vi "dfd_CIC Decimation Simu.vi"(0 "signal in":i32[](array[numeric]), 1 "lag":i32, 2 "#stage":i32, 3 "init? (T)":bool, 5 "factor":i32, 7 "Acc width":i32[](array[numeric]), 9 "MSB pos":i16, 11 "FXPMRateSimState in":T1, 12 "Output wl":i16, 13 "q_mode":T3=enum."Truncation" caption="rounding mode", 14 "phase":i32) -> (4 "signal out":i32[](array[numeric]), 15 "FXPMRateSimState out":T1)   [LabVIEW 2017, in "NI_DigFilter_FXP.lvlib"]
uses:
  <vilib>/addons/Digital Filter Design/NI_DigFilter_FXP.lvlib
  <vilib>/addons/Digital Filter Design/_Objects.llb/DFD Round-off Mode.ctl
  <vilib>/addons/Digital Filter Design/_Objects.llb/dfd_FXP MRate Simu State.ctl
  <vilib>/addons/Digital Filter Design/_Objects.llb/dfd_Integer I160.ctl
  <vilib>/addons/Digital Filter Design/NI_DigFilterLicensed.lvlib
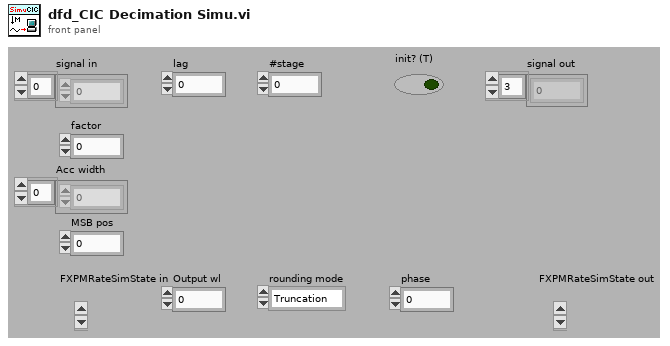
[diagram p1: front panel]
types:
  T1 = typedef "dfd_FXP MRate Simu State.ctl" = cluster{"acc1":T2[], "acc2":T2[], "FIR state":i64[], "next phase":i32}
  T2 = typedef "dfd_Integer I160.ctl" = cluster{"Hi [I32]":i32, "Lo3 [U32]":u32, "Lo2 [U32]":u32, "Lo1 [U32]":u32, "Lo0 [U32]":u32}
  T3 = typedef "NI_DigFilterLicensed.lvlib/DFD Round-off Mode.ctl" = enum16{"Nearest", "Truncation"}
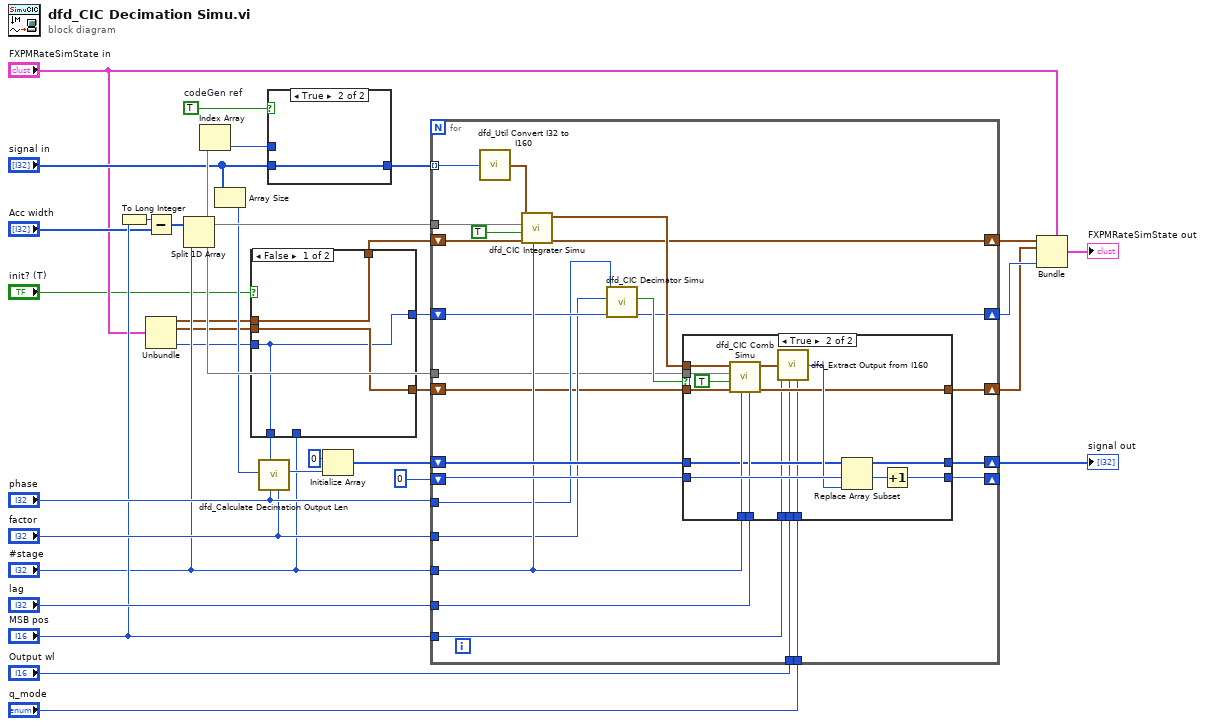
[diagram p0: block diagram]
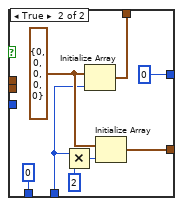
[diagram p2: hidden frame]
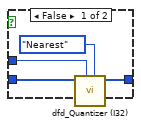
[diagram p3: hidden frame]
diagram:
  w12 = TRUE  # codeGen ref
  n1 = To Long Integer(number="MSB pos") -> (32bit integer=w19:i32)
  n2 = Subtract(x=w19, y="Acc width") -> (x-y=w16:i32[])
  n3 = Unbundle("FXPMRateSimState in") -> ("acc1"=w9:T2[], "acc2"=w8:T2[], "next phase"=w7:i32)  [unwired: 1 out]
  n4 = Split 1D Array(array=w16, index="#stage") -> (first subarray=w21:i32[], second subarray=w22:i32[])
  n5 = Index Array(array=w21) -> (element=w15:i32)  [unwired: 1 in]
  n6 = Array Size(array="signal in") -> (size(s)=w11:i32)
  n7 = case shown="False" "init? (T)" {
    tunnel: [w38 w46] -> w30
    tunnel: [w36 0] -> w29
    tunnel: [w37 w42] -> w28
    tunnel: "#stage" -> [_ w41]
    tunnel: [w36 0] -> w10
    tunnel: w9 -> [w38 _]
    tunnel: w8 -> [w37 _]
    tunnel: w7 -> [w36 _]
    frame False {
    }
    frame True {
      w43 = T2 {"Hi [I32]"=0, "Lo3 [U32]"=0, "Lo2 [U32]"=0, "Lo1 [U32]"=0, "Lo0 [U32]"=0} ("x [I160]")
      n8 = Multiply(x=w41, y=2) -> (x*y=w44:i32)
      n9 = Initialize Array(w43, w41) -> (w46:T2[])
      n10 = Initialize Array(w43, w44) -> (w42:T2[])
    }
  }
  n11 = call <vilib>:"dfd_Calculate Decimation Output Len.vi"("factor"="factor", "output phase"="phase", "current phase"=w10, "signal in len"=w11) -> ("signal out len"=w25:i32)  [unwired: 7 out]
  n12 = case shown="True" w12 {
    tunnel: w15 -> [w49 _]
    tunnel: "signal in" -> [w48 w51]
    tunnel: [w47 w51] -> w13
    frame False {
      n13 = call <vilib>:"dfd_Quantizer (I32).vi"("q_mode"=DFD_Round-off_Mode."Nearest", "LSB pos"=w49, "I32 in"=w48) -> ("I32 out"=w47:i32[])  [unwired: 8 out]
    }
    frame True {
    }
  }
  n14 = Initialize Array(0 ("element"), w25) -> (w34:i32[])
  n15 = for {
    tunnel: "#stage" -> [w69]
    tunnel: "factor" -> [w60]
    tunnel: "phase" -> [w59]
    tunnel: w13 -> [w70] mode=indexing
    shift-right: [w74] -> w32
    shift-left: w34 -> [w75]
    shift-right: [w72] -> _
    shift-left: 0 ("element") -> [w73]
    tunnel: "MSB pos" -> [w66]
    tunnel: "lag" -> [w71]
    shift-right: [w64] -> w3
    shift-left: w30 -> [w65]
    shift-right: [w61] -> w4
    shift-left: w29 -> [w62]
    shift-right: [w57] -> w2
    shift-left: w28 -> [w58]
    tunnel: "Output wl" -> [w56]
    tunnel: "q_mode" -> [w55]
    tunnel: w21 -> [w54]
    tunnel: w22 -> [w53]
    n16 = call <vilib>:"dfd_Util Convert I32 to I160.vi"("x [I32]"=w70) -> ("x [I160]"=w63:T2)  [unwired: 8 out]
    n17 = call <vilib>:"dfd_CIC Integrater Simu.vi"("stage"=w69, "acc in"=w65, "Decimation?"=TRUE, "Bit to cut"=w54, "x"=w63) -> ("acc out"=w64:T2[], "y"=w67:T2)  [unwired: 1 in, 4 out]
    n18 = call <vilib>:"dfd_CIC Decimator Simu.vi"("cnt in"=w62, "factor"=w60, "phase"=w59) -> ("cnt out"=w61:i32, "data valid?"=w68:bool)  [unwired: 2 in, 5 out]
    n19 = case shown="True" w68 {
      tunnel: w69 -> [_ w89]
      tunnel: w75 -> [w78 w84]
      tunnel: [w78 w93] -> w74
      tunnel: w73 -> [w77 w91]
      tunnel: [w77 w92] -> w72
      tunnel: w71 -> [_ w88]
      tunnel: w67 -> [_ w90]
      tunnel: w66 -> [_ w83]
      tunnel: w58 -> [w76 w86]
      tunnel: [w76 w85] -> w57
      tunnel: w56 -> [_ w82]
      tunnel: w55 -> [_ w81]
      tunnel: w53 -> [_ w80]
      frame False {
      }
      frame True {
        n20 = call <vilib>:"dfd_CIC Comb Simu.vi"("lag"=w88, "#stage"=w89, "history in"=w86, "Decimation?"=TRUE, "Bit to cut"=w80, "x"=w90) -> ("history out"=w85:T2[], "y"=w94:T2)  [unwired: 1 in, 3 out]
        n21 = call <vilib>:"dfd_Extract Output from I160.vi"("I160"=w94, "output MSB pos"=w83, "Output wl"=w82, "q_mode"=w81) -> ("y"=w87:i32)  [unwired: 5 out]
        n22 = Replace Array Subset(array=w84, new element=w87, index=w91) -> (w93:i32[])
        n23 = Increment(x=w91) -> (x+1=w92:i32)
      }
    }
  }
  "signal out" <- w32
  n24 = Bundle(cluster="FXPMRateSimState in", "acc1"=w3, "acc2"=w2, "next phase"=w4) -> (→"FXPMRateSimState out":T1)  [unwired: 1 out]
